vi "fftw_malloc_real_double.vi"(8 "error in (no error)":errorcluster, 11 "double count":u32=256) -> (0 "error out":errorcluster, 3 "*data":u64)   [LabVIEW 2020, in "FFTWDLL.lvlib"]
doc: "Allocate FFTW memory aligned for SIMD in double."
uses:
  FFTWDLL.lvlib
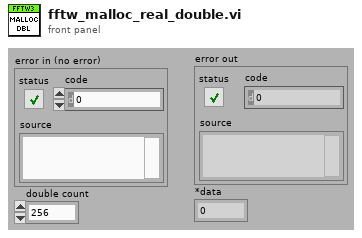
[diagram p1: front panel]
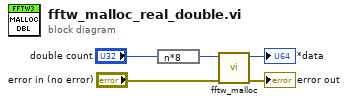
[diagram p0: block diagram]
diagram:
  n1 = expression code="n*8"("double count") -> (w4:u32)
  n2 = call "fftw_malloc.vi"("error in (no error)"="error in (no error)", "bytes count"=w4) -> ("error out"=→"error out":errorcluster, "*data"=→"*data":u64)  [unwired: 8 in]
